vi "Update Sys Def by Target type.vi"(7 "nodepaths":string[](array[string]), 8 "error in (no error)":errorcluster, 10 "Sys Def relative path:":path, 11 "VeriStandTestCase in":refnum<class "VeriStandTestCase.lvclass">) -> (0 "error out":errorcluster, 3 "VeriStandTestCase out":refnum<class "VeriStandTestCase.lvclass">)   [LabVIEW 2018]
doc: "This VI is used to update System Definition File based on specific Target Settings."
uses:
  niveristand-custom-device-testing-tools-master/VeriStandTestCase/VeriStandTestCase.lvclass
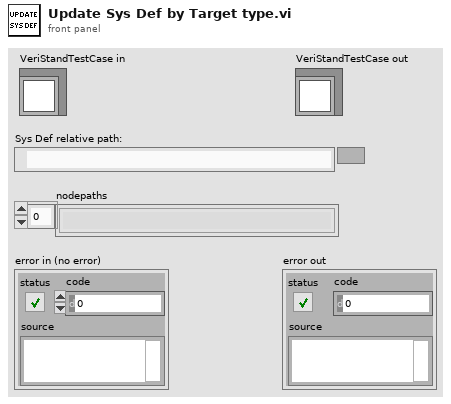
[diagram p1: front panel]
types:
  T1 = typedef "VeriStandTestUtilities.lvlib/TargetPlatform.ctl" = enum16{"Windows", "Linux64CRIO", "Linux64PXI", "LinuxARM", "PharLap"}
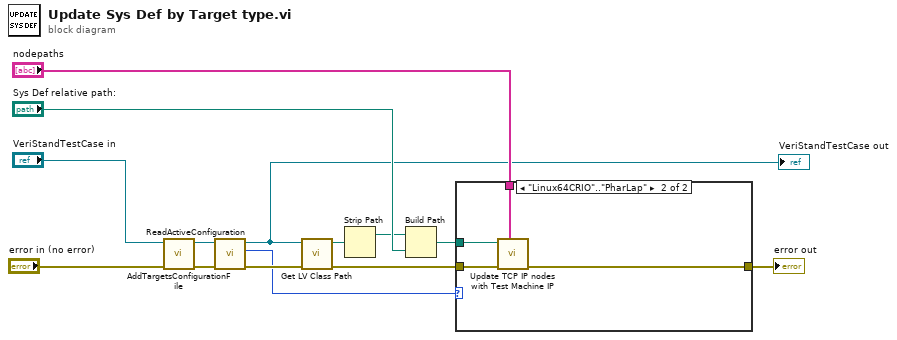
[diagram p0: block diagram]
diagram:
  n1 = call "AddTargetsConfigurationFile.vi"("error in (no error)"="error in (no error)", "VeriStandTestCase in"="VeriStandTestCase in") -> ("error out"=w4:errorcluster, "VeriStandTestCase out"=w2:refnum<class "VeriStandTestCase.lvclass">)  [unwired: 8 in]
  n2 = call-dynamic "ReadActiveConfiguration.vi"("error in (no error)"=w4, "VeriStandTestCase in"=w2) -> ("error out"=w11:errorcluster, "Target Platform"=w5:T1, "VeriStandTestCase out"=w7:refnum<class "VeriStandTestCase.lvclass">)  [unwired: 7 in]
  "VeriStandTestCase out" <- w7
  n3 = call <vilib>:"Get LV Class Path.vi"("error in (no error)"=w11, "object"=w7) -> ("error out"=w12:errorcluster, "class path"=w8:path)  [unwired: 8 in]
  n4 = Strip Path(path=w8) -> (stripped path=w9:path)  [unwired: 1 out]
  n5 = Build Path(base path=w9, name or relative path="Sys Def relative path:") -> (appended path=w13:path)
  n6 = case shown="\"Linux64CRIO\"..\"PharLap\"" w5 {
    tunnel: w12 -> [w15 w19]
    tunnel: [w15 w18] -> w6
    tunnel: w13 -> [_ w16]
    tunnel: "nodepaths" -> [_ w17]
    frame "Windows" {
    }
    frame "Linux64CRIO".."PharLap" {
      n7 = call "Update TCP IP nodes with Test Machine IP.vi"("nodepaths"=w17, "error in (no error)"=w19, "SysDef path in"=w16) -> ("error out"=w18:errorcluster)  [unwired: 7 in, 1 out]
    }
  }
  "error out" <- w6
